vi "Write Response to Stream.vi"(7 "Close? (T)":bool=TRUE, 8 "error in (no error)":errorcluster, 9 "Stream in":refnum<k5>, 11 "Streamable Response in":refnum<class "Streamable Response.lvclass">) -> (0 "error out":errorcluster, 3 "Streamable Response out":refnum<class "Streamable Response.lvclass">)   [LabVIEW 2020, in "HTTP Utils.lvlib" / "Streamable Response.lvclass"]
uses:
  Streamable Response.lvclass
  Streamable Response.lvclass/Streamable Response.ctl
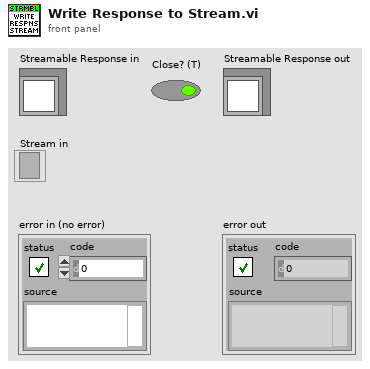
[diagram p1: front panel]
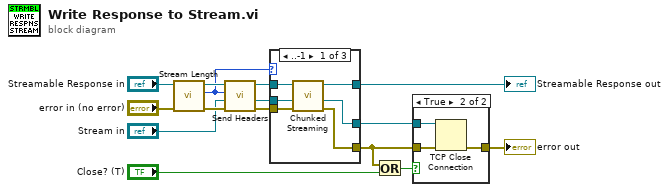
[diagram p0: block diagram]
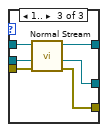
[diagram p3: hidden frame]
diagram:
  n1 = call-dynamic "Stream Length.vi"("error in (no error)"="error in (no error)", "Streamable Response in"="Streamable Response in") -> ("error out"=w9:errorcluster, "Stream Length"=w8:i64, "Streamable Response out"=w10:refnum<class "Streamable Response.lvclass">)  [unwired: 7 in]
  n2 = call "Send Headers.vi"("error in (no error)"=w9, "Stream in"="Stream in", "Content-Length"=w8, "Streamable Response in"=w10) -> ("error out"=w5:errorcluster, "Stream out"=w4:refnum<k5>, "Streamable Response out"=w6:refnum<class "Streamable Response.lvclass">)  [unwired: 5 in]
  n3 = case shown="..-1" w8 {
    tunnel: w5 -> [w19 w22 w25]
    tunnel: w6 -> [w20 w24 w27]
    tunnel: [w18 w23 w28] -> w12
    tunnel: [w17 w24 w30] -> w13
    tunnel: [w21 w22 w29] -> w2
    tunnel: w4 -> [w16 w23 w26]
    frame ..-1 {
      # "Unknown size, used chunked transfer which can send until done."
      n4 = call "Chunked Streaming.vi"("error in (no error)"=w19, "Stream in"=w16, "Streamable Response in"=w20) -> ("error out"=w21:errorcluster, "Stream out"=w18:refnum<k5>, "Streamable Response out"=w17:refnum<class "Streamable Response.lvclass">)  [unwired: 6 in]
    }
    frame 0 {
      # "No payload, just send headers"
    }
    frame 1.. {
      # "Normal streaming, send segments at a time."
      n5 = call "Normal Stream.vi"("error in (no error)"=w25, "Stream in"=w26, "Streamable Response in"=w27) -> ("error out"=w29:errorcluster, "Stream out"=w28:refnum<k5>, "Streamable Response out"=w30:refnum<class "Streamable Response.lvclass">)  [unwired: 6 in]
    }
  }
  "Streamable Response out" <- w13
  n6 = Or(x=w2, y="Close? (T)") -> (x .or. y?=w3:bool)
  n7 = case shown="True" w3 {
    tunnel: w2 -> [w31 w33]
    tunnel: w12 -> [_ w34]
    tunnel: [w31 w32] -> w11
    frame False {
    }
    frame True {
      n8 = TCP Close Connection(connection ID=w34, error in (no error)=w33) -> (error out=w32:errorcluster)  [unwired: 1 in, 1 out]
    }
  }
  "error out" <- w11
